vi "Pre Launch Init.vi"(11 "Nested in":refnum<class "APG.lvclass">) -> (0 "error out":errorcluster, 3 "Nested out":refnum<class "APG.lvclass">)   [LabVIEW 2021, in "APG.lvclass"]
doc: "(<B>Filename</B>: Actor Framework.lvlib:Actor.lvclass:Pre Launch Init.vi)\n\nDefines behavior that occurs after the Launch Nested Actor method is invoked but before the actor's Actor Core method begins running.\n\nBy default, this method does nothing. A descendant class may override it to define behavior."
uses:
  APG.lvclass
  APG.lvclass/APG.ctl
  <vilib>/MGI/Panel Manager/Panel Actor/Panel Actor/Panel Actor.lvclass
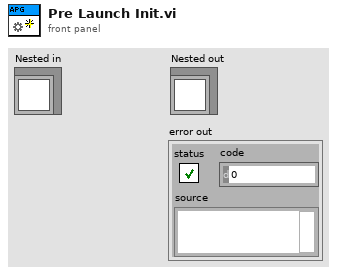
[diagram p1: front panel]
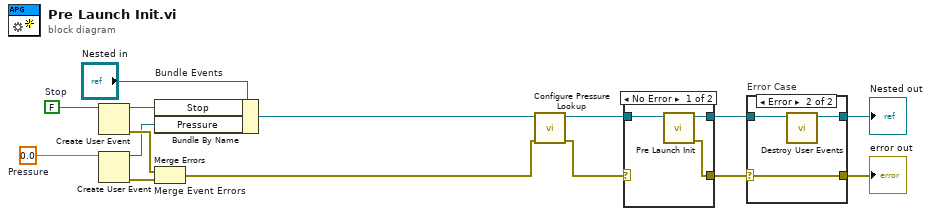
[diagram p0: block diagram]
diagram:
  w7 = 0.0  # Pressure
  w14 = FALSE  # Stop
  n1 = Create User Event(user event datatype=w14) -> (user event=w11:refnum<user-event>, error out=w13:errorcluster)  [unwired: 1 in]
  n2 = Create User Event(user event datatype=w7) -> (user event=w6:refnum<user-event>, error out=w5:errorcluster)  [unwired: 1 in]
  n3 = Bundle By Name "Bundle Events"(cluster="Nested in", "Stop"=w11, "Pressure"=w6) -> (w4:refnum<class "APG.lvclass">)
  n4 = Merge Errors "Merge Event Errors"(w13, w5) -> (w2:errorcluster)
  n5 = call "Configure Pressure Lookup.vi"("error in (no error)"=w2, "APG in"=w4) -> ("error out"=w1:errorcluster, "APG out"=w3:refnum<class "APG.lvclass">)  [unwired: 8 in]
  n6 = case shown="No Error" w1 {
    selector: w1 -> [_ w20]
    tunnel: [w18 w19] -> w9
    tunnel: w3 -> [w17 w19]
    tunnel: [w16 w20] -> w8
    frame No Error {
      n7 = call-parent "Pre Launch Init.vi"("Panel Actor in"=w17) -> ("error out"=w16:errorcluster, "Panel Actor out"=w18:refnum<class "APG.lvclass">)  [unwired: 9 in]
    }
    frame Error {
    }
  }
  n8 = case "Error Case" shown="Error" w8 {
    selector: w8 -> [w21 w25]
    tunnel: w9 -> [w22 w24]
    tunnel: [w22 w23] -> w12
    tunnel: [w21 w25] -> w10
    frame No Error {
    }
    frame Error {
      n9 = call "Destroy User Events.vi"("UI Template in"=w24) -> ("UI Template out"=w23:refnum<class "APG.lvclass">)  [unwired: 10 in]
    }
  }
  "error out" <- w10
  "Nested out" <- w12
